vi "CG test stand analog read.vi"() -> ()   [LabVIEW 2020]
doc: "This example demonstrates how to read N channels of analog input from a LINX device."
uses:
  <vilib>/MakerHub/LINX/Public/Peripherals/Analog/Analog Read N Chans.vi
  <vilib>/MakerHub/LINX/Private/Local IO/LinxAnalogRead.vi
  <vilib>/MakerHub/LINX/Public/Utilities/Check Channel.vi
  <vilib>/MakerHub/LINX/Public/Utilities/Open Serial.vi
  <vilib>/MakerHub/LINX/Private/Utilties/Generate Error.vi
  <vilib>/MakerHub/LINX/LMH-LINX.lvlib
panel:
  out "Calibrated value":dbl
  in  "B":dbl
  in  "A":dbl
  in  "Analog Port":dbl
  out "Time Stamp":timestamp
  out "Input data":dbl(graph)
  out "Voltage":dbl
  in  "Stop Button":bool
  out "Loop Rate (Hz)":u32
  in  "Serial Port":refnum<visa-resource-name>
  # "X"
  # "+"
  # "Analog Read N Channels Example (Serial Interface)\n\nThis example demonstrates how to read N channels of analog input values from a LINX device connected to the host computer via Serial / USB.\n\nInstructions\n1. Select the COM Port associated with the LINX Device.\n2. Select the Analog Channels to read.\n3. Click the Run Arrow."
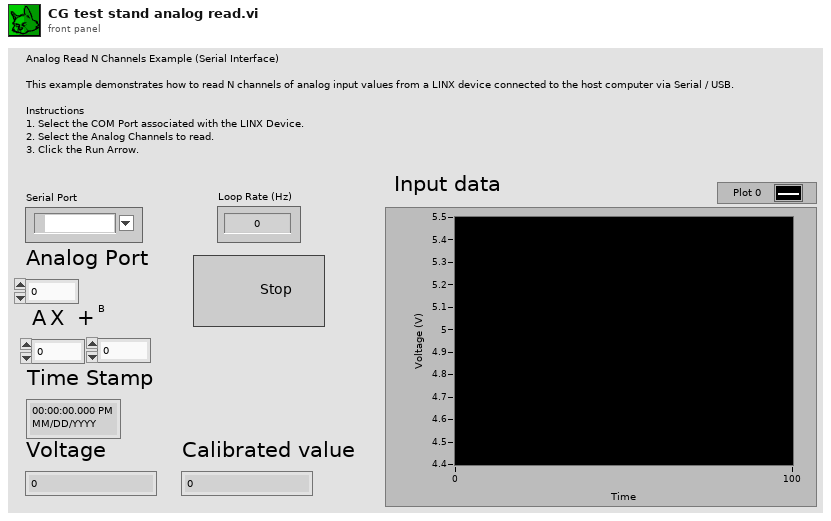
[diagram p1: front panel]
types:
  T1 = typedef "LMH-LINX.lvlib/LINX Ref.ctl" = cluster{"IO":T2, "Interface":T3, "LINX Device Config":T4}
  T2 = typedef "LMH-LINX.lvlib/Platform.ctl" = enum16{"Remote", "Local"}
  T3 = typedef "LMH-LINX.lvlib/Interface.ctl" = enum16{"Serial", "TCP"}
  T4 = typedef "LMH-LINX.lvlib/Device.lvlib/LINX Device Config.ctl" = cluster{"Interface":T3, "COM Port":refnum<visa-resource-name>, "TCP Configuration":T5, "Device Family":u8, "Device ID":u8, "Device Name":string, "TCP Ref":refnum<k5>, "Channels":T6}
  T5 = typedef "LMH-LINX.lvlib/Device.lvlib/TCP Config.ctl" = cluster{"IP Address":string, "Port":u16}
  T6 = typedef "LMH-LINX.lvlib/Channels.ctl" = cluster{"DI":u8[], "DO":u8[], "AI":u8[], "AO":u8[], "PWM":u8[], "QE":u8[], "UART":u8[], "I2C 2":u8[], "SPI":u8[], "CAN":u8[], "Servo":u8[], "AI Ref (V)":dbl, "AI Resolution (Bits)":u8, "AO Ref (V)":dbl, "AO Resolution (Bits)":u8}
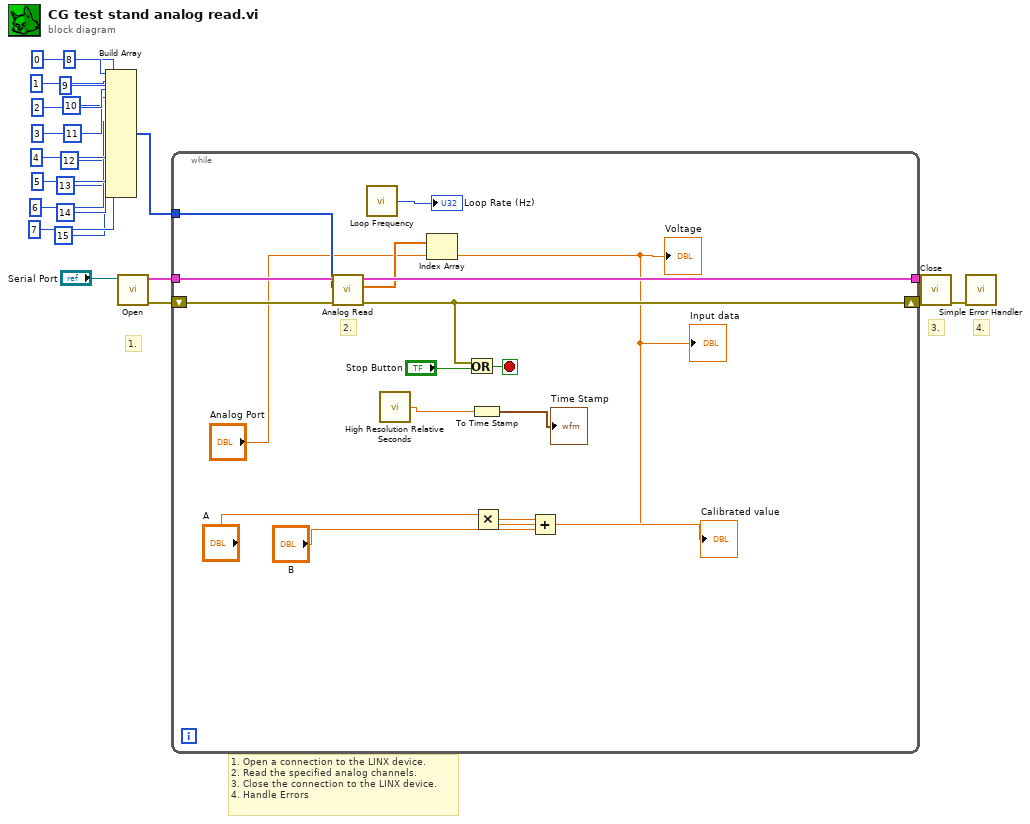
[diagram p0: block diagram]
diagram:
  # "1. Open a connection to the LINX device.\n2. Read the specified analog channels.\n3. Close the connection to the LINX device.\n4. Handle Errors"
  # "4."
  # "3."
  # "1."
  n1 = Build Array(0, 1, 2, 3, 4, 5, 6, 7, 8, 9, 10, 11, 12, 13, 14, 15) -> (w17:i32[])
  n2 = call-poly <vilib>:"Open.vi"("Serial Port"="Serial Port") -> ("Error Out"=w22:errorcluster, "LINX Resource"=w23:T1)  [unwired: 8 in, 1 out]
  n3 = while {
    tunnel: w23 -> [w40]
    tunnel: [w38] -> w21
    shift-right: [w35] -> w20
    shift-left: w22 -> [w39]
    tunnel: w17 -> [w34]
    stop <- w37 stop-if-true
    # "2."
    n4 = call-poly <vilib>:"Analog Read.vi"("Error In"=w39, "AI Channel(s)"=w34, "LINX Resource"=w40) -> ("Error Out"=w35:errorcluster, "Voltages"=w33:dbl[], "LINX Resource"=w38:T1)  [unwired: 5 in, 1 out]
    n5 = call <vilib>:"Loop Frequency.vi"() -> ("Loop Rate (Hz)"=→"Loop Rate (Hz)":u32)
    n6 = call <vilib>:"High Resolution Relative Seconds.vi"() -> ("relative seconds"=w32:dbl)
    n7 = Index Array(array=w33, index="Analog Port") -> (element=w24:dbl)
    "Voltage" <- w24
    "Input data" <- w24
    n8 = Or(x=w35, y="Stop Button") -> (x .or. y?=w37:bool)
    n9 = To Time Stamp(1:w32) -> (0:→"Time Stamp":timestamp)
    n10 = Multiply(x="A", y=w24) -> (x*y=w28:dbl)
    n11 = Add(x=w28, y="B") -> (x+y=→"Calibrated value":dbl)
  }
  n12 = call <vilib>:"Close.vi"("Error In"=w20, "LINX Resource"=w21) -> ("Error Out"=w18:errorcluster)  [unwired: 9 in]
  n13 = call <vilib>:"Simple Error Handler.vi"("error in (no error)"=w18) -> ()  [unwired: 4 in, 5 out]
